vi "Pre Launch Init.vi"(11 "Engine in":refnum<class "Engine.lvclass">) -> (0 "error out":errorcluster, 3 "Engine out":refnum<class "Engine.lvclass">)   [LabVIEW 2023, in "Engine.lvlib" / "Engine.lvclass"]
doc: "Initializes the Engine Actor. \n\nThis calls create references, call parent method, then concludes with Initialize.\n\nThis guarantees that error management queues, report queues and any other necessary references are created as needed."
uses:
  Library/Engine.lvclass
  builds/Framework/Panel Manager.lvlibp/Library/Panel Actor.lvclass
  Library/Engine.lvclass/Engine.ctl
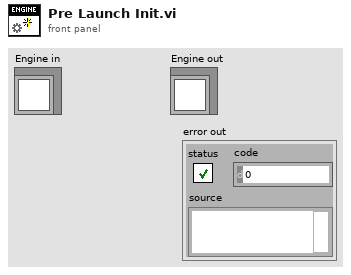
[diagram p1: front panel]
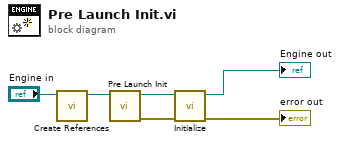
[diagram p0: block diagram]
diagram:
  n1 = call "Create References.vi"("Engine in"="Engine in") -> ("Engine out"=w1:refnum<class "Engine.lvclass">)  [unwired: 9 in, 1 out]
  n2 = call-parent "Pre Launch Init.vi"("Panel Actor in"=w1) -> ("error out"=w5:errorcluster, "Panel Actor out"=w6:refnum<class "Engine.lvclass">)  [unwired: 9 in]
  n3 = call-dynamic "Initialize.vi"("error in (no error)"=w5, "Engine in"=w6) -> ("error out"=→"error out":errorcluster, "Engine out"=→"Engine out":refnum<class "Engine.lvclass">)  [unwired: 8 in]
